vi "运维调试_总磷总氮.vi"() -> ()   [LabVIEW 2016, in "斯坦道仪器.lvlib"]
uses:
  <vilib>/Platform/TimedLoop/XDataNode/timing_clust.ctl
  <vilib>/Platform/TimedLoop/XDataNode/nitl_modes.ctl
  <vilib>/Platform/TimedLoop/XDataNode/wakeup.ctl
  <vilib>/Utility/miscctls.llb/LVPointTypeDef.ctl
  <vilib>/Utility/config.llb/Read Key (Double).vi
  <vilib>/Utility/config.llb/Write Key (Double).vi
  <vilib>/Platform/TimedLoop/XDataNode/XDataNode.xnode
  <vilib>/Platform/TimedLoop/XDataNode/XDNodeRunTimeDep.lvlib
  <vilib>/Utility/config.llb/NI_LVConfig.lvlib
panel:
  in  "返回 2":bool
  in  "设置 2":bool
  out "总氮稀释倍数":dbl
  out "固件版本号":string
  in  "数组":string[](array[string])
  in  "备用系数写入":bool
  in  "备用系数读取":bool
  in  "备用系数":T1
  in  "量程切换阈值写入":bool
  in  "量程切换阈值读取":bool
  in  "量程切换阈值":cluster{"阈值":dbl, "标液浓度":dbl}
  in  "参数下拉列表":enum16{"总磷", "总氮"}(ring)
  in  "量程下拉列表":enum16{"低量程", "高量程"}(ring)
  in  "测量模式下拉列表":enum16{"水样测量", "空白核查", "跨度核查", "标样核查", "加标回收"}(ring)
  in  "公式":cluster{"X^2":dbl, "X":dbl, "b":dbl}
  in  "写公式":bool
  in  "读公式":bool
  in  "精度":dbl=4.0
  in  "样品5 F0":dbl
  in  "样品5 F1":dbl
  in  "样品4 F1":dbl
  in  "样品4 F0":dbl
  in  "样品3 F0":dbl
  in  "样品3 F1":dbl
  in  "样品2 F0":dbl
  in  "样品2 F1":dbl
  in  "样品1 F1":dbl
  in  "样品1 F0":dbl
  in  "method":u16(ring) items=["最小二乘", "最小绝对残差", "Bisquare"]
  in  "模型":enum32{"线性", "多项式"}(ring)
  out "r^2":dbl format="%.7g"
  out "拟合公式":string
  in  "样品2启用":bool
  in  "样品5启用":bool
  in  "样品4启用":bool
  in  "样品3启用":bool
  in  "样品1启用":bool
  in  "标液浓度5":dbl
  in  "测量吸光度5":dbl
  in  "标液浓度4":dbl
  in  "测量吸光度4":dbl
  in  "标液浓度3":dbl
  in  "测量吸光度3":dbl
  in  "标液浓度2":dbl
  in  "测量吸光度2":dbl
  in  "测量吸光度1":dbl
  in  "标液浓度1":dbl
  out "XY图":cluster{"X Values":dbl[], "Y Values":dbl[]}[](graph)
  in  "返回":bool
  in  "调试":bool
  out "序列号":string="序列号"
  out "总氮测量数据":T2(xcontrol)
  out "总磷测量数据":T2(xcontrol)
  out "集成报警信息":string
  out "设置值":dbl
  out "定时启动":bool
  out "总磷总氮运行状态":T3(xcontrol)
  in  "停止":bool
  in  "手动启动":bool
  in  "单步测试":bool
  in  "总磷氨氮调试":u16[](xcontrol)
  out "F3":sgl format="%#.6f"
  out "F2":sgl format="%#.6f"
  out "F1":sgl format="%#.6f"
  out "F0":sgl format="%#.6f"
  out "多列列表框":i32(listbox)
  # "COM5"
  # "参数设置"
  # "标液浓度"
  # "F0"
  # "F1"
  # "吸光值显示"
  # "辅\n助\n计\n算\n区"
  # "样品一"
  # "样品二"
  # "样品三"
  # "样品四"
  # "样品五"
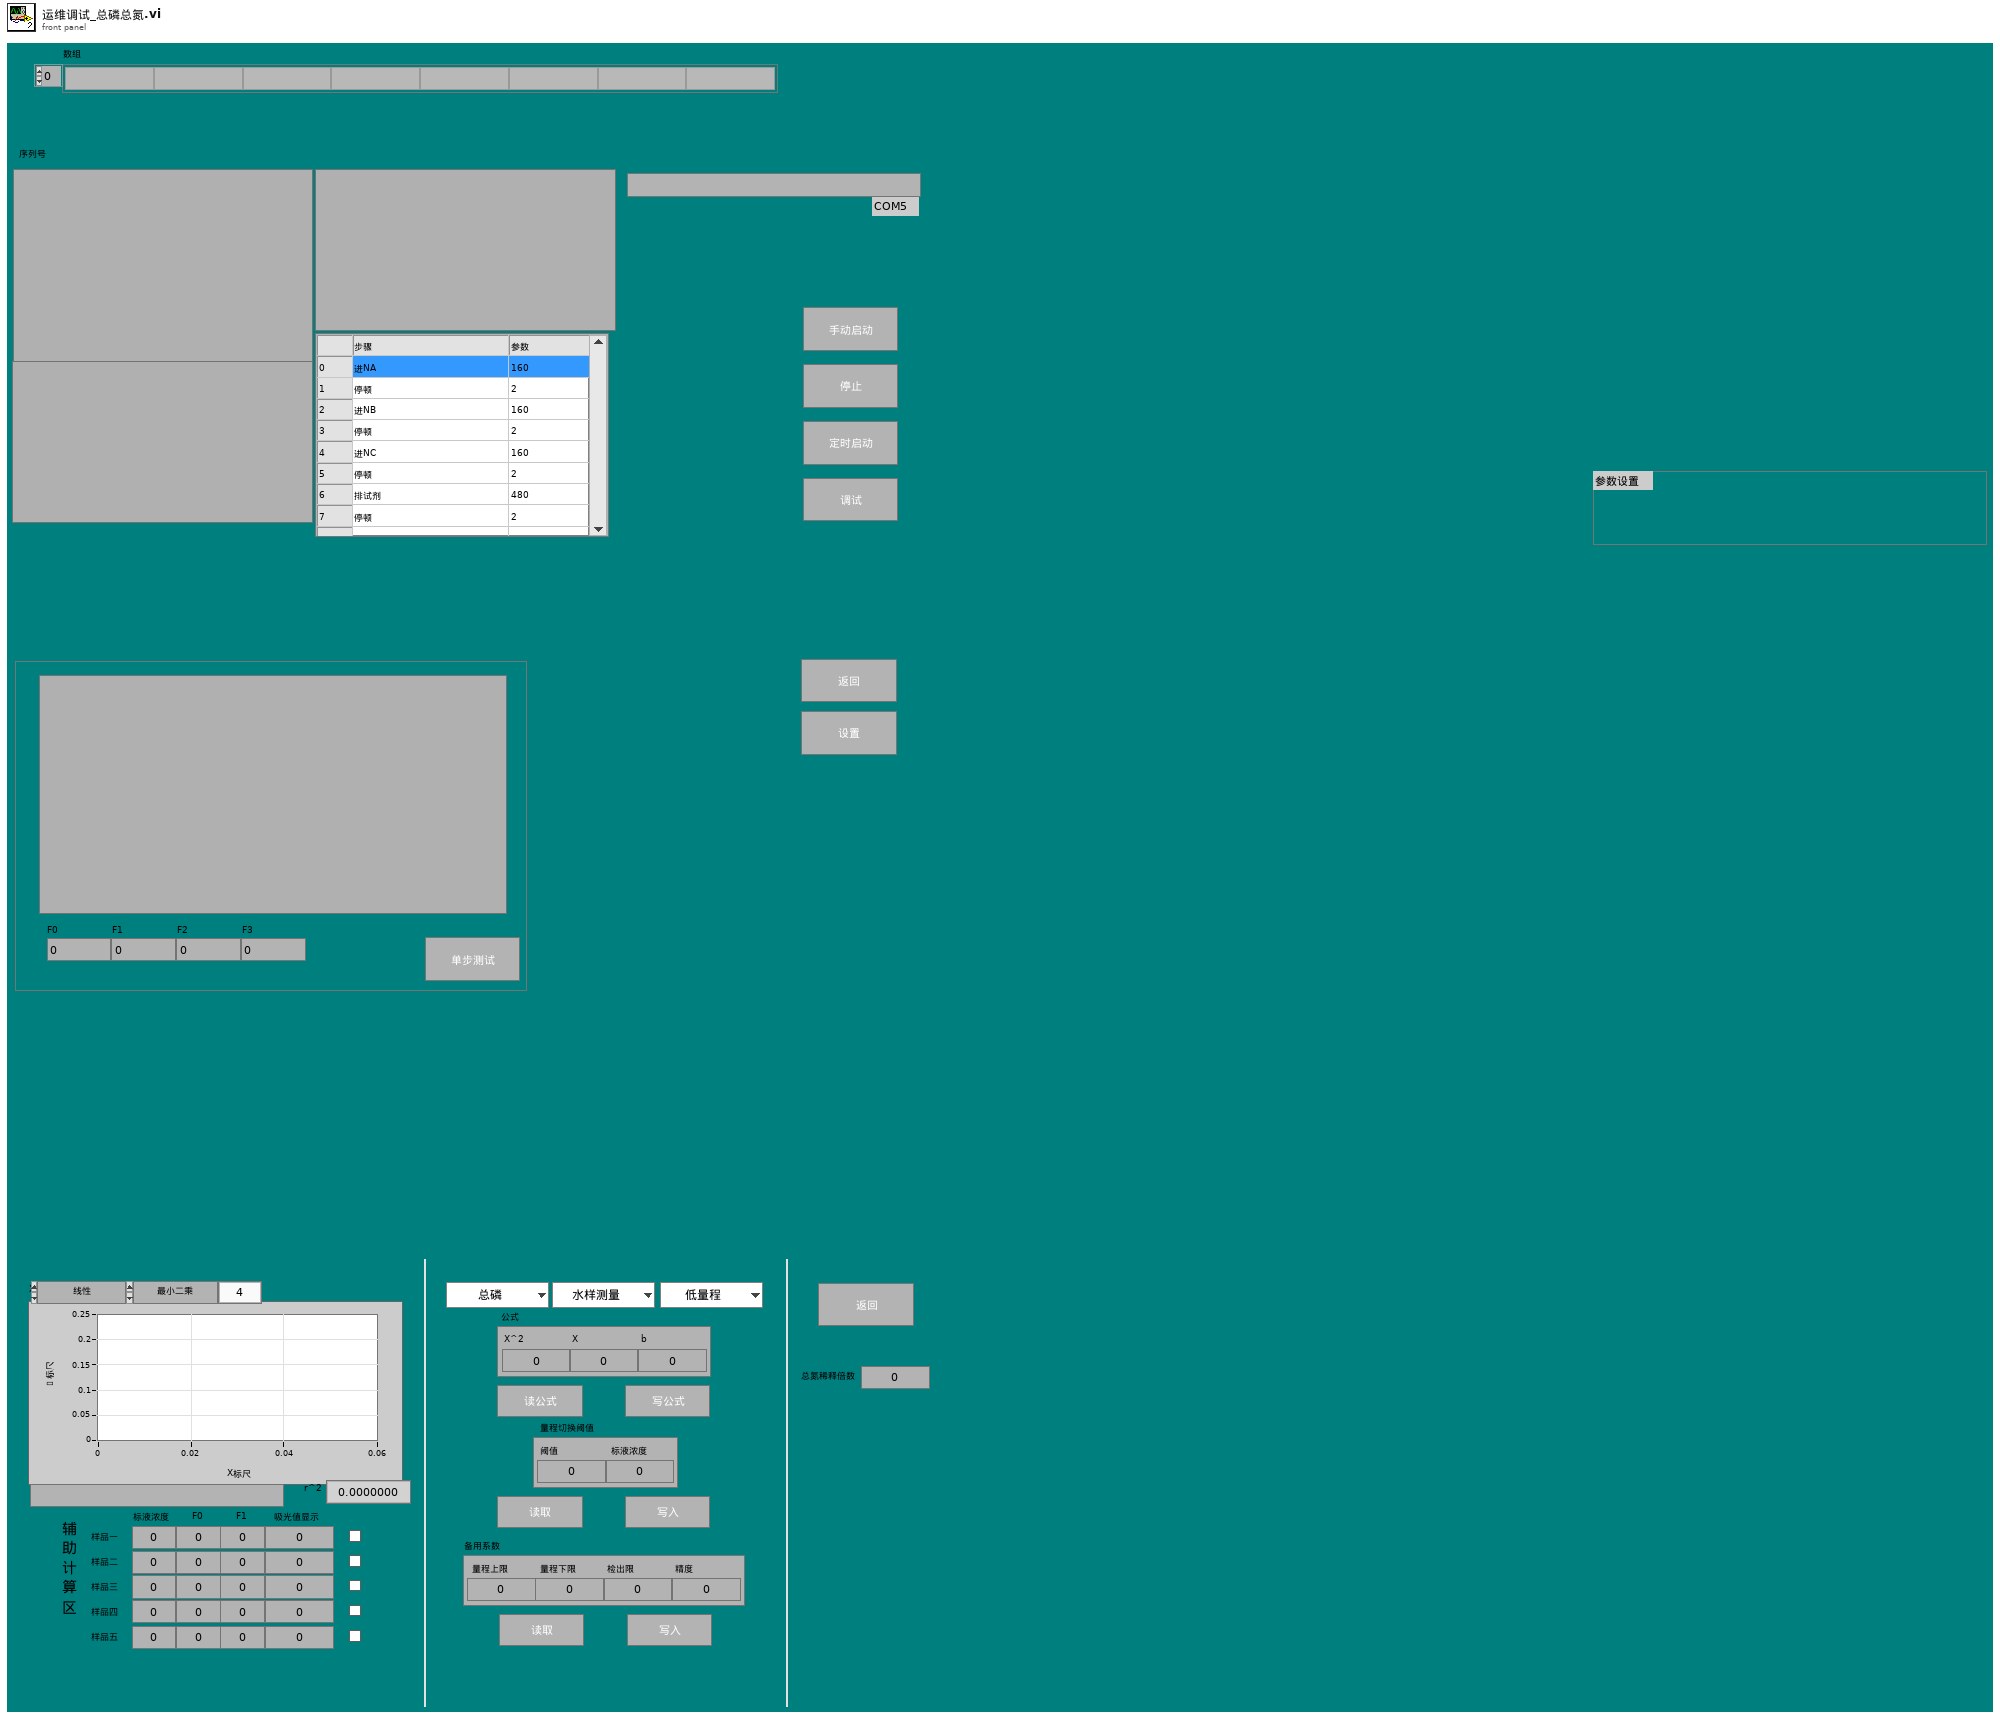
[diagram p1: front panel]
types:
  T1 = cluster{"量程上限":dbl, "量程下限":dbl, "检出限":dbl, "精度":dbl}
  T2 = cluster{"flowid":u16, "测量精度":u16, "测量数据区":cluster{"因子编码":u32, "单位":u16, "标样参考值":sgl, "水样数据时间":timestamp, "水样实测值":sgl, "水样数据标识":string, "标样数据时间":timestamp, "标样实测值":sgl, "标样数据标识":string, "空白数据时间":timestamp, "空白实测值":sgl, "空白数据标识":string, "零点核查数据时间":timestamp, "零点核查实测值":sgl, "零点核查数据标识":string, "跨度核查数据时间":timestamp, "跨度核查实测值":sgl, "跨度核查数据标识":string, "加标回收数据时间":timestamp, "加标回收实测值":sgl, "加标回收数据标识":string, "平行样数据时间":timestamp, "平行样实测值":sgl, "平行样数据标识":string, "F0":sgl, "F1":sgl, "F2":sgl, "F3":sgl, "F4":sgl, "F5":sgl, "F6":sgl, "F7":sgl, "温度":sgl, "湿度":sgl, "X值":sgl}}
  T3 = cluster{"系统时间":timestamp, "工作状态":enum16{"空闲", "水样测试", "标样核查", "零点核查", "跨度核查", "空白测试", "平行样测试", "加标回收", "空白校准", "标样校准", "初始化（清洗）"}, "测量模式":enum16{"待机", "连续模式", "周期模式", "定点模式", "受控模式", "手动模式"}, "告警代码":enum16{"无告警", "缺试剂告警", "缺水样告警", "缺蒸馏水告警", "缺标液告警", "仪表漏液告警", "标定异常告警", "超量程告警", "加热异常", "低试剂预警", "超上限告警", "超下限告警", "仪表内部其他异常", "滴定异常告警", "电极异常告警", "量程切换告警", "参数设置告警", "PH电极电位异常", "电导率电极异常", "浊度光度异常", "溶解氧电极异常", "溶解氧光强异常", "温度异常告警", "PH异常告警", "溶解氧异常告警", "电导率异常告警", "浊度异常告警", "叶绿素异常告警", "藻密度异常告警", "蓝绿藻异常告警", "ORP异常告警", "氨氮异常告警", "清洁刷异常告警", "SD卡异常告警", "蓝牙异常告警", "Wifi异常告警", "流程异常告警"}, "故障代码":enum16{"无故障", "电机故障", "温度故障", "通讯故障", "滴定故障"}, "日志代码":u16, "软件版本":u16, "F0":sgl, "F1":sgl, "F2":sgl, "F3":sgl, "T":sgl, "H":sgl, "id":u16, "flowid":u16, "量程":u16}
  T4 = enum16{"待机", "启动氨氮", "氨氮测量中", "启动总磷", "总磷测量中", "延时"}
  T5 = typedef "LVPointTypeDef.ctl" = cluster{"Horizontal":i16, "Vertical":i16}
  T6 = cluster{"因子编码":u32, "单位":u16, "标样参考值":sgl, "水样数据时间":timestamp, "水样实测值":sgl, "水样数据标识":string, "标样数据时间":timestamp, "标样实测值":sgl, "标样数据标识":string, "空白数据时间":timestamp, "空白实测值":sgl, "空白数据标识":string, "零点核查数据时间":timestamp, "零点核查实测值":sgl, "零点核查数据标识":string, "跨度核查数据时间":timestamp, "跨度核查实测值":sgl, "跨度核查数据标识":string, "加标回收数据时间":timestamp, "加标回收实测值":sgl, "加标回收数据标识":string, "平行样数据时间":timestamp, "平行样实测值":sgl, "平行样数据标识":string, "F0":sgl, "F1":sgl, "F2":sgl, "F3":sgl, "F4":sgl, "F5":sgl, "F6":sgl, "F7":sgl, "温度":sgl, "湿度":sgl, "X值":sgl}
  T7 = enum16{"空闲", "水样测试", "标样核查", "零点核查", "跨度核查", "空白测试", "平行样测试", "加标回收", "空白校准", "标样校准", "初始化（清洗）"}
  T8 = typedef "XDNodeRunTimeDep.lvlib/timing_clust.ctl" = cluster{"Expected End [f-1]":u64, "Actual End [f-1]":u64, "Finished Late? [f-1]":bool, "Expected End [i-1]":u64, "Actual End [i-1]":u64, "Finished Late? [i-1]":bool, "Expected Start [i]":u64, "Actual Start [i]":u64, "Expected Start [f]":u64, "Actual Start [f]":u64, "Source Name":string, "Structure Name":string, "Period":i64, "Deadline":i64, "Offset":i64, "Start":i64, "Priority":i32, "Timeout":i32, "Mode":T9, "Wakeup Reason":T10, "Error":errorcluster, "Source Type":string, "Secondary Source Type":string, "Global End Time":u64, "Global Start Time":u64, "Frame Duration":u64, "Iteration Duration":u64, "Assigned CPU":i32, "I/O Scan Engine Mode":u32}
  T9 = typedef "XDNodeRunTimeDep.lvlib/nitl_modes.ctl" = enum32{"No Change", "Process missed periods, maintain original phase", "Discard missed periods, maintain original phase", "Process missed periods, ignore original phase", "Discard missed periods, ignore original phase"}
  T10 = typedef "XDNodeRunTimeDep.lvlib/wakeup.ctl" = enum32{"Normal", "Aborted", "Asynchronous wakeup", "Timing source error", "Timed loop error", "Timeout"}
  T11 = cluster{"启动模式":enum16{"标液测量", "水样测量", "零液测量", "盲样测量", "加标回收"}, "启动参数":u16, "量程":enum16{"低量程", "高量程"}}
  T12 = cluster{"时间标识":timestamp, "设备":string, "日志信息":string, "流程参数":string}
  T13 = cluster{"时间标识":timestamp, "设备":string, "日志信息":string}
  T14 = enum16{"无告警", "缺试剂告警", "缺水样告警", "缺蒸馏水告警", "缺标液告警", "仪表漏液告警", "标定异常告警", "超量程告警", "加热异常", "低试剂预警", "超上限告警", "超下限告警", "仪表内部其他异常", "滴定异常告警", "电极异常告警", "量程切换告警", "参数设置告警", "PH电极电位异常", "电导率电极异常", "浊度光度异常", "溶解氧电极异常", "溶解氧光强异常", "温度异常告警", "PH异常告警", "溶解氧异常告警", "电导率异常告警", "浊度异常告警", "叶绿素异常告警", "藻密度异常告警", "蓝绿藻异常告警", "ORP异常告警", "氨氮异常告警", "清洁刷异常告警", "SD卡异常告警", "蓝牙异常告警", "Wifi异常告警", "流程异常告警"}
  T15 = typedef "LVRowAndColumnUnsignedTypeDef.ctl" = cluster{"Row":u32, "Column":u32}
  T16 = typedef "NI_LVConfig.lvlib/Config Data RefNum.ctl" = refnum<k1>
  T17 = cluster{"站号":u16, "量程切换":enum32{"H", "L", "AUTO"}, "控制命令":enum16{"启动测量", "标样核查", "零点核查", "跨度核查", "空白测试", "平行样测试", "加标回收", "空白校准", "标样校准", "初始化（清洗）", "停止测试", "仪器重启", "校时", "模式设置", "测量间隔设置", "盲样测试"}, "模式设置":enum16{"待机", "连续模式", "周期模式", "定点模式", "受控模式", "手动模式"}, "测量间隔":u16}
  T18 = cluster{"站号":u16, "量程切换":enum32{"H", "L", "AUTO"}, "控制命令":enum16{"启动测量", "标样核查", "零点核查", "跨度核查", "空白测试", "平行样测试", "加标回收", "空白校准", "标样校准", "初始化（清洗）", "停止测试", "仪器重启", "校时", "模式设置", "测量间隔设置"}, "模式设置":enum16{"待机", "连续模式", "周期模式", "定点模式", "受控模式", "手动模式"}, "测量间隔":u16}
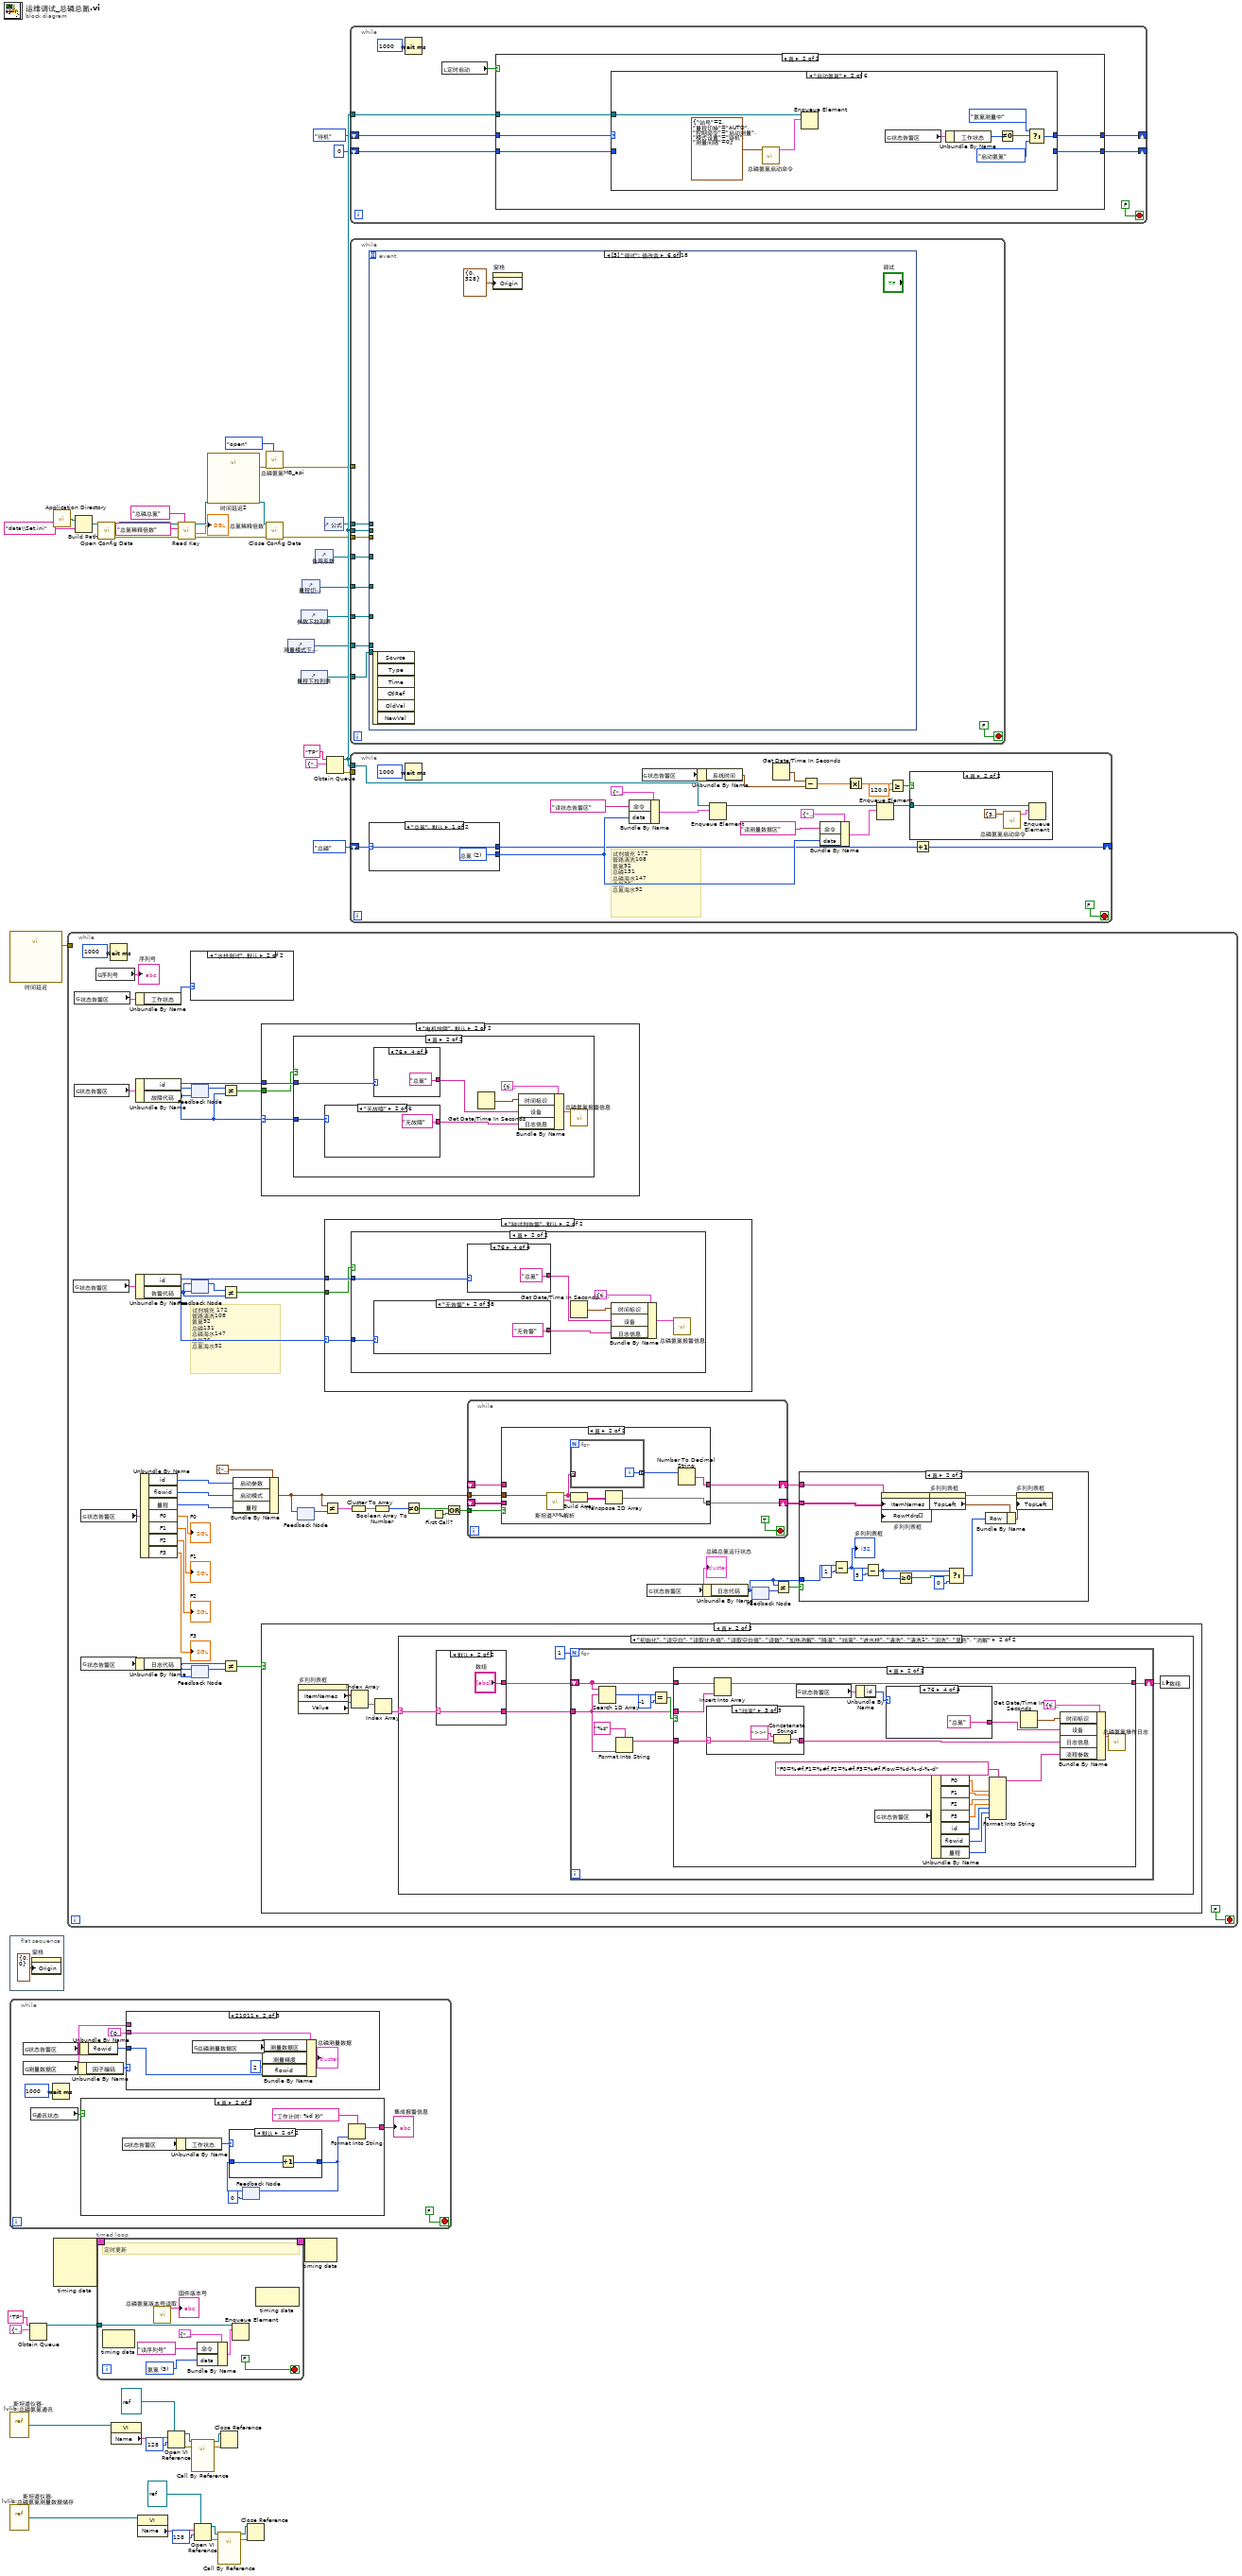
[diagram p0: block diagram]
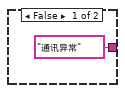
[diagram p2: hidden frame]
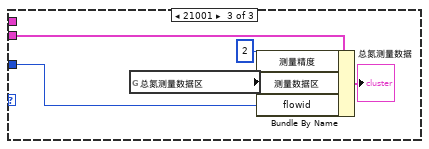
[diagram p5: hidden frame]
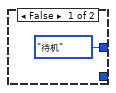
[diagram p6: hidden frame]
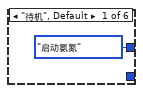
[diagram p7: hidden frame]
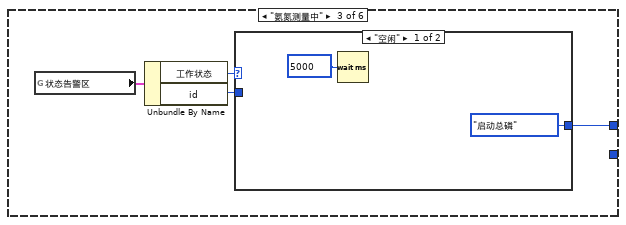
[diagram p8: hidden frame]
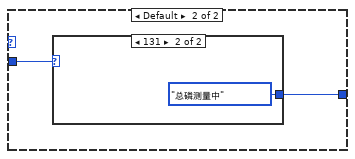
[diagram p9: hidden frame]
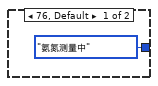
[diagram p10: hidden frame]
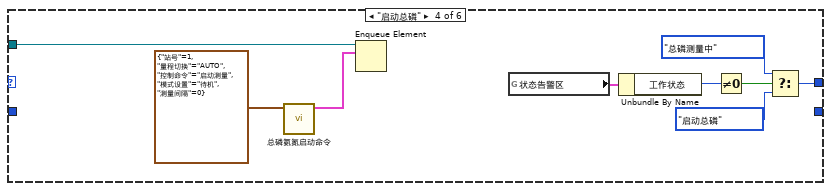
[diagram p11: hidden frame]
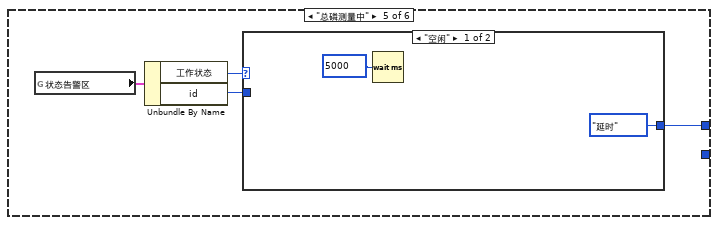
[diagram p12: hidden frame]
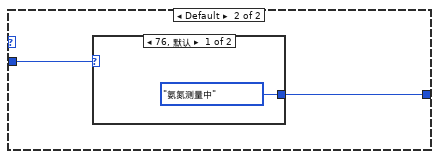
[diagram p13: hidden frame]
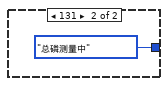
[diagram p14: hidden frame]
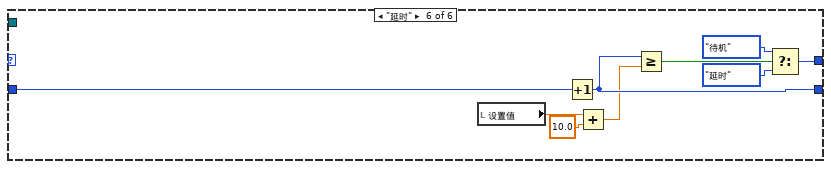
[diagram p15: hidden frame]
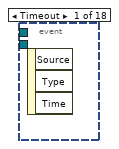
[diagram p16: hidden frame]
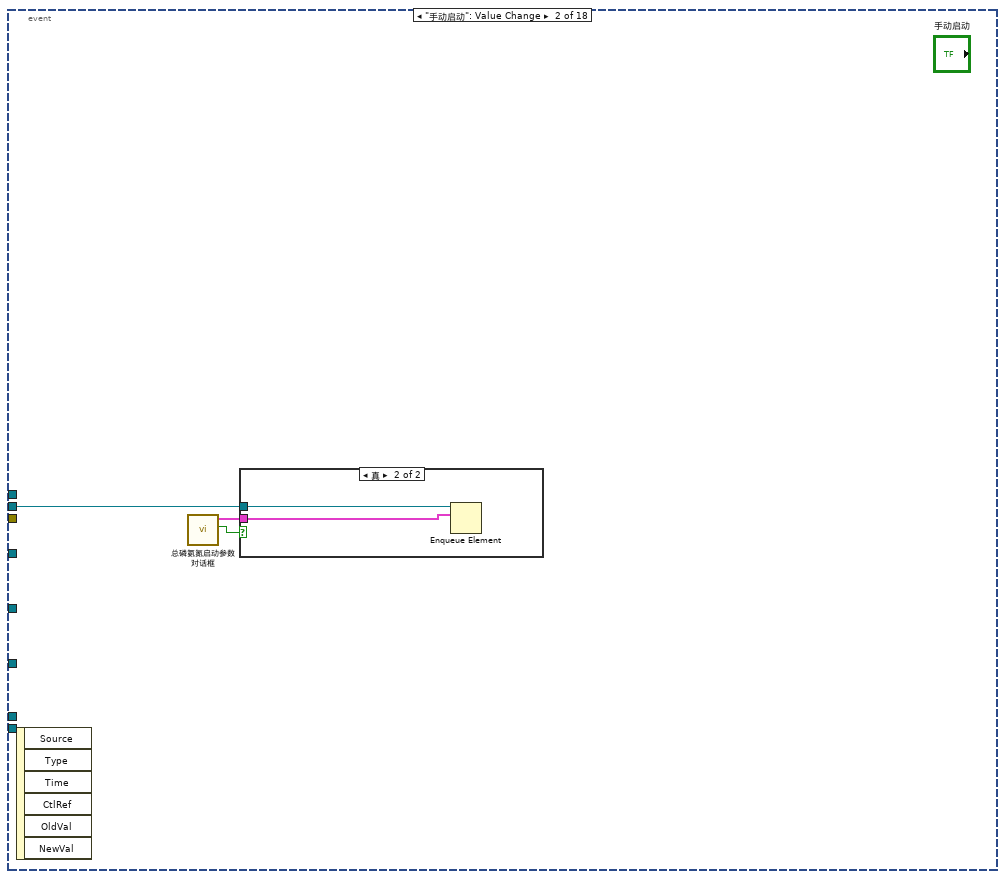
[diagram p17: hidden frame]
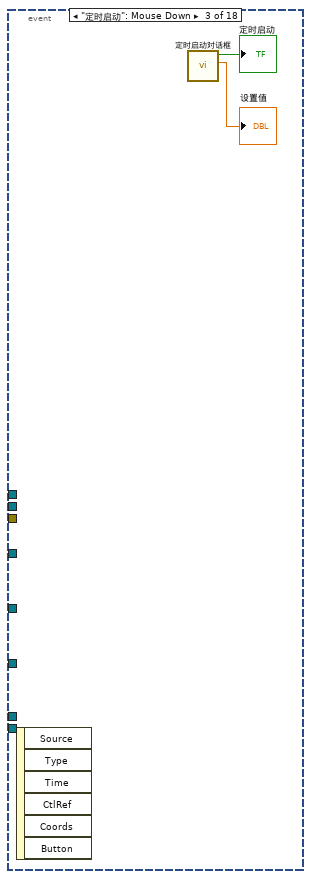
[diagram p19: hidden frame]
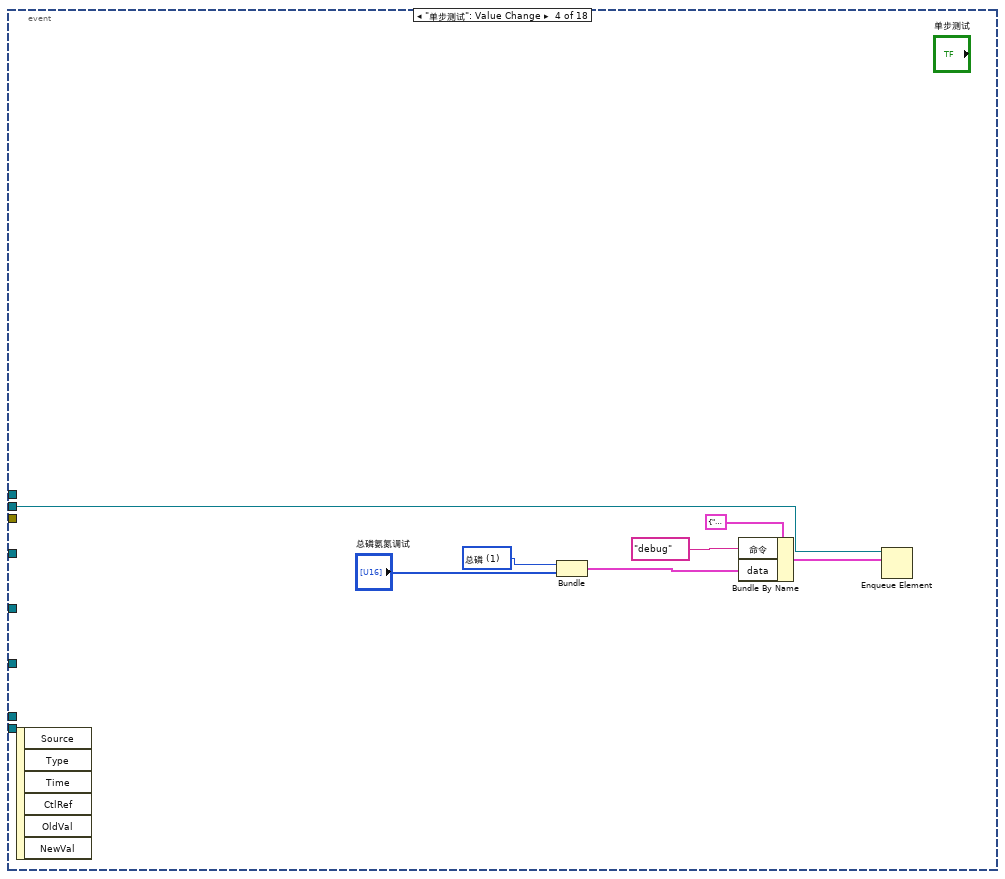
[diagram p20: hidden frame]
diagram:
  n1 = call "时间延迟"() -> ("error out"=w20:errorcluster)  [unwired: 11 in]
  n2 = flat-sequence {
    frame #0 {
      n3 = property on="窗格" class="Pane"("Origin"=T5 {"Horizontal"=0, "Vertical"=0} ("原点")) -> ()  [unwired: 2 in, 2 out]
    }
  }
  n4 = while {
    stop <- FALSE stop-if-true
    n5 = global read "VAR总磷氨氮全局变量.vi" "状态告警区"() -> (w53:T3)
    n6 = global read "VAR总磷氨氮全局变量.vi" "测量数据区"() -> (w57:T6)
    n7 = global read "VAR总磷氨氮全局变量.vi" "通讯状态"() -> (w55:bool)
    n8 = Wait (ms)(milliseconds to wait=u32 1000 ("等待时间（毫秒）")) -> ()  [unwired: 1 out]
    n9 = Unbundle By Name(w57) -> ("因子编码"=w56:u32)
    n10 = Unbundle By Name(w53) -> ("flowid"=w52:u16)
    n11 = case shown="真" w55 {
      tunnel: ["通讯异常" ("集成报警信息") w61] -> w54
      frame False {
      }
      frame True {
        n12 = global read "VAR总磷氨氮全局变量.vi" "状态告警区"() -> (w67:T3)
        n13 = Unbundle By Name(w67) -> ("工作状态"=w66:T7)
        n14 = feedback #1(0) -> (w64:i32)
        n15 = case shown="默认" w66 {
          tunnel: w64 -> [_ w69]
          tunnel: [_ w68] -> w62
          frame "空闲" {
          }
          frame Default {
            n16 = Increment(x=w69) -> (x+1=w68:i32)
          }
        }
        n17 = feedback-in #1(w62) -> ()
        n18 = Format Into String(format string="工作计时: %d 秒" ("格式字符串"), w62) -> (resulting string=w61:string)  [unwired: 2 in, 1 out]
      }
    }
    "集成报警信息" <- w54
    n19 = case shown="21011" w56 {
      tunnel: w57 -> [_ _ _]
      tunnel: w52 -> [_ w72 w78]
      tunnel: T2 {"flowid"=0, "测量精度"=0, "测量数据区"={"因子编码"=0, "单位"=0, "标样参考值"=0.0, "水样数据时间"=timestamp(0 s since 1904-01-01), "水样实测值"=0.0, "水样数据标识"="", "标样数据时间"=timestamp(0 s since 1904-01-01), "标样实测值"=0.0, "标样数据标识"="", "空白数据时间"=timestamp(0 s since 1904-01-01), "空白实测值"=0.0, "空白数据标识"="", "零点核查数据时间"=timestamp(0 s since 1904-01-01), "零点核查实测值"=0.0, "零点核查数据标识"="", "跨度核查数据时间"=timestamp(0 s since 1904-01-01), "跨度核查实测值"=0.0, "跨度核查数据标识"="", "加标回收数据时间"=timestamp(0 s since 1904-01-01), "加标回收实测值"=0.0, "加标回收数据标识"="", "平行样数据时间"=timestamp(0 s since 1904-01-01), "平行样实测值"=0.0, "平行样数据标识"="", "F0"=0.0, "F1"=0.0, "F2"=0.0, "F3"=0.0, "F4"=0.0, "F5"=0.0, "F6"=0.0, "F7"=0.0, "温度"=0.0, "湿度"=0.0, "X值"=0.0}} ("总氮测量数据") -> [_ w71 w77]
      frame Default {
      }
      frame 21011 {
        n20 = global read "VAR总磷氨氮全局变量.vi" "总磷测量数据区"() -> (w70:T6)
        n21 = Bundle By Name(cluster=w71, "测量数据区"=w70, "测量精度"=u16 2, "flowid"=w72) -> (→"总磷测量数据":T2)
      }
      frame 21001 {
        n22 = global read "VAR总磷氨氮全局变量.vi" "总氮测量数据区"() -> (w75:T6)
        n23 = Bundle By Name(cluster=w77, "测量精度"=u16 2, "测量数据区"=w75, "flowid"=w78) -> (→"总氮测量数据":T2)
      }
    }
  }
  n24 = vi-ref "斯坦道仪器.lvlib:总磷氨氮通讯.vi"() -> (w43:refnum<vi>)
  n25 = vi-ref "斯坦道仪器.lvlib:总磷氨氮测量数据储存.vi"() -> (w35:refnum<vi>)
  n26 = Obtain Queue(name (unnamed)="TP" ("名称（未命名）"), element data type=cluster{"命令":string, "data":variant} {"命令"="", "data"=variant}) -> (queue out=w13:refnum<queue>)  [unwired: 3 in, 2 out]
  n27 = node-c288() -> (w17:T8)  [unwired: 4 in]
  n28 = call <vilib>:"Application Directory.vi"() -> ("Application Directory"=w7:path)
  n29 = while {
    tunnel: w20 -> [_]
    stop <- FALSE stop-if-true
    # "试剂填充 172 \n管路清洗108\n氨氮92\n总磷131\n总磷海水147\n总氮76\n总氮海水92"
    n30 = global read "VAR总磷氨氮全局变量.vi" "状态告警区"() -> (w96:T3)
    n31 = global read "VAR总磷氨氮全局变量.vi" "状态告警区"() -> (w91:T3)
    n32 = global read "VAR总磷氨氮全局变量.vi" "状态告警区"() -> (w85:T3)
    n33 = global read "VAR总磷氨氮全局变量.vi" "状态告警区"() -> (w108:T3)
    n34 = global read "VAR总磷氨氮全局变量.vi" "状态告警区"() -> (w82:T3)
    n35 = global read "VAR总磷氨氮全局变量.vi" "序列号"() -> (→"序列号":string)
    n36 = Wait (ms)(milliseconds to wait=u32 1000 ("等待时间（毫秒）")) -> ()  [unwired: 1 out]
    n37 = Unbundle By Name(w85) -> ("工作状态"=w84:T7)
    n38 = Unbundle By Name(w91) -> ("id"=w90:u16, "故障代码"=w87:enum16{"无故障", "电机故障", "温度故障", "通讯故障", "滴定故障"})
    n39 = Unbundle By Name(w96) -> ("id"=w95:u16, "告警代码"=w92:T14)
    n40 = Unbundle By Name(w82) -> ("日志代码"=w81:u16)
    n41 = Unbundle By Name(w108) -> ("id"=w105:u16, "flowid"=w107:u16, "量程"=w106:u16, "F0"=→"F0":sgl, "F1"=→"F1":sgl, "F2"=→"F2":sgl, "F3"=→"F3":sgl)
    n42 = case shown="\"水样测试\", 默认" w84 {
      frame "空闲" {
        n43 = local write "数组"(string[] [] ("数组")) -> ()
      }
      frame "水样测试", Default {
      }
    }
    n44 = feedback #2(w87) -> (w88:enum16{"无故障", "电机故障", "温度故障", "通讯故障", "滴定故障"})
    n45 = feedback-in #2(w87) -> ()
    n46 = feedback #3(w92) -> (w93:T14)
    n47 = feedback-in #3(w92) -> ()
    n48 = feedback #4(w81) -> (w83:u16)
    n49 = feedback-in #4(w81) -> ()
    n50 = Not Equal?(x=w88, y=w87) -> (x != y?=w89:bool)
    n51 = Not Equal?(x=w93, y=w92) -> (x != y?=w94:bool)
    n52 = Not Equal?(x=w81, y=w83) -> (x != y?=w80:bool)
    n53 = Bundle By Name(cluster=T11 {"启动模式"=enum."加标回收", "启动参数"=1, "量程"=enum."低量程"} ("参数簇"), "启动参数"=w105, "启动模式"=w107, "量程"=w106) -> (w98:T11)
    n54 = case shown="\"电机故障\", 默认" w87 {
      selector: w87 -> [_ w177]
      tunnel: w90 -> [_ w178]
      tunnel: w89 -> [_ w176]
      frame "无故障" {
      }
      frame "电机故障", Default {
        n55 = case shown="真" w176 {
          tunnel: w178 -> [_ w185]
          tunnel: w177 -> [_ w180]
          frame False {
          }
          frame True {
            n56 = case shown="\"无故障\"" w180 {
              selector: w180 -> [w187 _ _ _ _ _]
              tunnel: [w186 "无故障" "电机故障" "温度故障" "通讯故障" "滴定故障"] -> w179
              frame Default {
                n57 = Format Into String(format string="%d" ("格式字符串"), initial string="未知" ("工作状态"), w187) -> (resulting string=w186:string)  [unwired: 1 in, 1 out]
              }
              frame "无故障" {
              }
              frame "电机故障" {
              }
              frame "温度故障" {
              }
              frame "通讯故障" {
              }
              frame "滴定故障" {
              }
            }
            n58 = case shown="76" w185 {
              tunnel: [_ "总磷" ("table输入") "氨氮" ("table输入") "总氮" ("table输入")] -> w181
              frame Default {
              }
              frame 131 {
              }
              frame 92 {
              }
              frame 76 {
              }
            }
            n59 = Get Date/Time In Seconds() -> (seconds since 1Jan1904=w182:timestamp)
            n60 = Bundle By Name(cluster=T13 {"时间标识"=timestamp(0 s since 1904-01-01), "设备"="", "日志信息"=""} ("data in"), "时间标识"=w182, "设备"=w181, "日志信息"=w179) -> (w183:T13)
            n61 = call "总磷氨氮报警信息.vi"("data in"=w183) -> ()  [unwired: 11 in]
          }
        }
      }
    }
    n62 = case shown="真" w80 {
      frame False {
      }
      frame True {
        n63 = property on="多列列表框" class="MCListbox (严格)"() -> ("ItemNames"=w125:string[][], "Value"=w126:i32)  [unwired: 2 in, 2 out]
        n64 = Index Array(array=w125, index (row)=w126) -> (element=w124:string[])  [unwired: 1 in]
        n65 = Index Array(array=w124) -> (element=w123:string)  [unwired: 1 in]
        n66 = case shown="\"初始化\", \"读空白\", \"读取比色值\", \"读取空白值\", \"读数\", \"加热消解\", \"降温\", \"结束\", \"进水样\", \"清洗\", \"清洗1\", \"润洗\", \"显色\", \"消解\"" w123 {
          selector: w123 -> [_ w129]
          frame Default {
          }
          frame "初始化", "读空白", "读取比色值", "读取空白值", "读数", "加热消解", "降温", "结束", "进水样", "清洗", "清洗1", "润洗", "显色", "消解" {
            n67 = case shown="默认" w129 {
              selector: w129 -> [w133 w135]
              tunnel: [w133 w135] -> w128
              tunnel: [string[] [] ("数组") "数组"] -> w127
              frame "读数" {
              }
              frame Default {
              }
            }
            n68 = for {
              N: 1 -> [_]
              tunnel: w128 -> [w137]
              shift-right: [w136] -> w130
              shift-left: w127 -> [w138]
              n69 = Search 1D Array(1D array=w138, element=w137) -> (index of element=w141:i32)  [unwired: 1 in]
              n70 = Format Into String(format string="%s" ("格式字符串"), w137) -> (resulting string=w142:string)  [unwired: 2 in, 1 out]
              n71 = Equal?(x=w141, y=-1) -> (x = y?=w139:bool)
              n72 = case shown="真" w139 {
                tunnel: w142 -> [_ w146]
                tunnel: w138 -> [w144 w150]
                tunnel: w137 -> [_ w149]
                tunnel: [w144 w148] -> w136
                frame False {
                }
                frame True {
                  n73 = case shown="\"结束\"" w146 {
                    selector: w146 -> [w166 w169 w172]
                    tunnel: [w166 w168 w171] -> w145
                    frame Default {
                    }
                    frame "初始化" {
                      n74 = Concatenate Strings("<<" ("字符串"), w169) -> (w168:string)
                    }
                    frame "结束" {
                      n75 = Concatenate Strings(">>" ("字符串"), w172) -> (w171:string)
                    }
                  }
                  n76 = Insert Into Array(array=w150, new element=w149) -> (w148:string[])  [unwired: 1 in]
                  n77 = global read "VAR总磷氨氮全局变量.vi" "状态告警区"() -> (w165:T3)
                  n78 = Unbundle By Name(w165) -> ("id"=w164:u16)
                  n79 = global read "VAR总磷氨氮全局变量.vi" "状态告警区"() -> (w160:T3)
                  n80 = case shown="76" w164 {
                    tunnel: [_ "总磷" ("table输入") "氨氮" ("table输入") "总氮" ("table输入")] -> w162
                    frame Default {
                    }
                    frame 131 {
                    }
                    frame 92 {
                    }
                    frame 76 {
                    }
                  }
                  n81 = Unbundle By Name(w160) -> ("F0"=w157:sgl, "F1"=w156:sgl, "F2"=w155:sgl, "F3"=w154:sgl, "id"=w153:u16, "flowid"=w152:u16, "量程"=w151:u16)
                  n82 = Format Into String(format string="F0=%#f,F1=%#f,F2=%#f,F3=%#f,Flow=%d-%-d-%-d" ("格式字符串"), w157, w156, w155, w154, w153, w152, w151) -> (resulting string=w158:string)  [unwired: 2 in, 1 out]
                  n83 = Get Date/Time In Seconds() -> (seconds since 1Jan1904=w161:timestamp)
                  n84 = Bundle By Name(cluster=T12 {"时间标识"=timestamp(0 s since 1904-01-01), "设备"="", "日志信息"="", "流程参数"=""} ("data in"), "时间标识"=w161, "设备"=w162, "日志信息"=w145, "流程参数"=w158) -> (w163:T12)
                  n85 = call "总磷氨氮操作日志.vi"("data in"=w163) -> ()  [unwired: 11 in]
                }
              }
            }
            n86 = local write "数组"(w130) -> ()
          }
        }
      }
    }
    n87 = feedback #5() -> (w114:T11)  [unwired: 1 in]
    n88 = feedback-in #5(w98) -> ()
    n89 = Not Equal?(x=w98, y=w114) -> (x != y?=w115:cluster{"启动模式":bool, "启动参数":bool, "量程":bool})
    n90 = case shown="\"缺试剂告警\", 默认" w92 {
      selector: w92 -> [_ w199]
      tunnel: w95 -> [_ w200]
      tunnel: w94 -> [_ w198]
      frame "无告警" {
      }
      frame "缺试剂告警", Default {
        n91 = case shown="真" w198 {
          tunnel: w200 -> [_ w207]
          tunnel: w199 -> [_ w201]
          frame False {
          }
          frame True {
            n92 = case shown="\"无告警\"" w201 {
              selector: w201 -> [w209 _ _ _ _ _ _ _ _ _ _ _ _ _ _ _ _ _ _ _ _ _ _ _ _ _ _ _ _ _ _ _ _ _ _ _ _ _]
              tunnel: [w208 "无告警" "缺试剂告警" "缺水样告警" "缺蒸馏水告警" "缺标液告警" "仪表漏液告警" "标定异常告警" "超量程告警" "加热异常" "低试剂预警" "超上限告警" "超下限告警" "仪表内部其他异常" "滴定异常告警" "电极异常告警" "量程切换告警" "参数设置告警" "PH电极电位异常" "电导率电极异常" "浊度光度异常" "溶解氧电极异常" "溶解氧光强异常" "温度异常告警" "PH异常告警" "溶解氧异常告警" "电导率异常告警" "浊度异常告警" "叶绿素异常告警" "藻密度异常告警" "蓝绿藻异常告警" "ORP异常告警" "氨氮异常告警" "清洁刷异常告警" "SD卡异常告警" "蓝牙异常告警" "WiFi异常告警" "流程异常告警"] -> w202
              frame Default {
                n93 = Format Into String(format string="%d" ("格式字符串"), initial string="未知" ("工作状态"), w209) -> (resulting string=w208:string)  [unwired: 1 in, 1 out]
              }
              frame "无告警" {
              }
              frame "缺试剂告警" {
              }
              frame "缺水样告警" {
              }
              frame "缺蒸馏水告警" {
              }
              frame "缺标液告警" {
              }
              frame "仪表漏液告警" {
              }
              frame "标定异常告警" {
              }
              frame "超量程告警" {
              }
              frame "加热异常" {
              }
              frame "低试剂预警" {
              }
              frame "超上限告警" {
              }
              frame "超下限告警" {
              }
              frame "仪表内部其他异常" {
              }
              frame "滴定异常告警" {
              }
              frame "电极异常告警" {
              }
              frame "量程切换告警" {
              }
              frame "参数设置告警" {
              }
              frame "PH电极电位异常" {
              }
              frame "电导率电极异常" {
              }
              frame "浊度光度异常" {
              }
              frame "溶解氧电极异常" {
              }
              frame "溶解氧光强异常" {
              }
              frame "温度异常告警" {
              }
              frame "PH异常告警" {
              }
              frame "溶解氧异常告警" {
              }
              frame "电导率异常告警" {
              }
              frame "浊度异常告警" {
              }
              frame "叶绿素异常告警" {
              }
              frame "藻密度异常告警" {
              }
              frame "蓝绿藻异常告警" {
              }
              frame "ORP异常告警" {
              }
              frame "氨氮异常告警" {
              }
              frame "清洁刷异常告警" {
              }
              frame "SD卡异常告警" {
              }
              frame "蓝牙异常告警" {
              }
              frame "Wifi异常告警" {
              }
              frame "流程异常告警" {
              }
            }
            n94 = case shown="76" w207 {
              tunnel: [_ "总磷" ("table输入") "氨氮" ("table输入") "总氮" ("table输入")] -> w203
              frame Default {
              }
              frame 131 {
              }
              frame 92 {
              }
              frame 76 {
              }
            }
            n95 = Get Date/Time In Seconds() -> (seconds since 1Jan1904=w204:timestamp)
            n96 = Bundle By Name(cluster=T13 {"时间标识"=timestamp(0 s since 1904-01-01), "设备"="", "日志信息"=""} ("data in"), "时间标识"=w204, "设备"=w203, "日志信息"=w202) -> (w205:T13)
            n97 = call "总磷氨氮报警信息.vi"("data in"=w205) -> ()  [unwired: 11 in]
          }
        }
      }
    }
    n98 = Cluster To Array(cluster=w115) -> (array=w116:bool[])
    n99 = Boolean Array To Number(Boolean array=w116) -> (number=w117:u32)
    n100 = Not Equal To 0?(x=w117) -> (x != 0?=w110:bool)
    n101 = First Call?() -> (First Call?: T/F=w111:bool)
    n102 = Or(x=w110, y=w111) -> (x .or. y?=w109:bool)
    n103 = while {
      tunnel: w109 -> [w258]
      tunnel: w98 -> [w257]
      shift-right: [w256] -> w113
      shift-left: _ -> [w252]
      shift-right: [w255] -> w112
      shift-left: _ -> [w253]
      stop <- TRUE stop-if-true
      n104 = case shown="真" w258 {
        tunnel: [w260 w267] -> w255
        tunnel: [w259 w266] -> w256
        tunnel: w257 -> [_ w261]
        tunnel: w253 -> [w260 _]
        tunnel: w252 -> [w259 _]
        frame False {
        }
        frame True {
          n105 = call "斯坦道XML解析.vi"("参数簇"=w261) -> ("步骤时间"=w262:string[], "步骤名"=w264:string[])  [unwired: 9 in]
          n106 = for {
            tunnel: w264 -> [_] mode=indexing
            tunnel: [w268] -> w265 mode=indexing
            i -> [w268]
          }
          n107 = Build Array(w264, w262) -> (w263:string[][])
          n108 = Transpose 2D Array(2D array=w263) -> (transposed array=w266:string[][])
          n109 = Number To Decimal String(number=w265) -> (decimal integer string=w267:string[])  [unwired: 1 in]
        }
      }
    }
    n110 = global read "VAR总磷氨氮全局变量.vi" "状态告警区"() -> (w99:T3)
    "总磷总氮运行状态" <- w99
    n111 = Unbundle By Name(w99) -> ("日志代码"=w86:u16)
    n112 = feedback-in #6(w86) -> ()
    n113 = feedback #6() -> (w119:u16)  [unwired: 1 in]
    n114 = Not Equal?(x=w86, y=w119) -> (x != y?=w118:bool)
    n115 = case shown="真" w118 {
      tunnel: w86 -> [_ w271]
      tunnel: w113 -> [_ w278]
      tunnel: w112 -> [_ w277]
      frame False {
      }
      frame True {
        n116 = Subtract(x=w271, y=1) -> (x-y=w269:i32)
        "多列列表框" <- w269
        n117 = Subtract(x=w269, y=5) -> (x-y=w273:i32)
        n118 = property on="多列列表框" class="MCListbox (严格)"("ItemNames"=w278, "RowHdrs[]"=w277) -> (error out=w279:errorcluster)  [unwired: 2 in, 1 out]
        n119 = Greater Or Equal To 0?(x=w273) -> (x >= 0?=w272:bool)
        n120 = property on="多列列表框" class="MCListbox (严格)"(error in=w279) -> (error out=w280:errorcluster, "TopLeft"=w281:T15)  [unwired: 1 in, 1 out]
        n121 = Select(t=w273, s=w272, f=0) -> (s? t:f=w274:i32)
        n122 = Bundle By Name(cluster=w281, "Row"=w274) -> (w282:T15)
        n123 = property on="多列列表框" class="MCListbox (严格)"(error in=w280, "TopLeft"=w282) -> ()  [unwired: 1 in, 2 out]
      }
    }
  }
  n124 = Build Path(base path=w7, name or relative path="data\\Set.ini" ("名称或相对路径")) -> (appended path=w5:path)
  n125 = timed-loop {
    timing: w17 -> [_]
    timing-out: [_] -> w16
    tunnel: w13 -> [w285]
    stop <- FALSE stop-if-true
    w286 = u16 3 items=["总磷"=1, "氨氮"=3] ("站号")
    # "定时更新"
    n126 = node-c288() -> ()  [unwired: 1 in, 1 out]
    n127 = call "总磷氨氮版本号读取.vi"() -> ("固件版本号"=→"固件版本号":string)  [unwired: 11 in]
    n128 = Bundle By Name(cluster=cluster{"命令":string, "data":variant} {"命令"="", "data"=variant} ("元素"), "命令"="读序列号", "data"=w286) -> (w284:cluster{"命令":string, "data":variant})
    n129 = Enqueue Element(queue=w285, element=w284) -> ()  [unwired: 2 in, 3 out]
    n130 = node-c288() -> ()  [unwired: 1 in, 1 out]
  }
  n131 = call <vilib>:"Open Config Data.vi"("configuration file path"=w5) -> ("error out"=w9:errorcluster, "refnum"=w11:T16)  [unwired: 8 in, 1 out]
  n132 = property class="VI"(reference=w43) -> ("Name"=w42:string)  [unwired: 1 in, 2 out]
  n133 = property class="VI"(reference=w35) -> ("Name"=w28:string)  [unwired: 1 in, 2 out]
  n134 = Open VI Reference(type specifier VI Refnum (for type only)=refnum<vi> refnum, vi path=w42, options=128 ("选项")) -> (vi reference=w40:refnum<vi>, error out=w38:errorcluster)  [unwired: 3 in]
  n135 = call-poly <vilib>:"Read Key.vi"("section"="总磷总氮", "error in (no error)"=w9, "key"="总氮稀释倍数" ("section"), "refnum"=w11) -> ("error out"=w8:errorcluster, "value"=→"总氮稀释倍数":dbl, "refnum out"=w10:T16)  [unwired: 4 in, 1 out]
  n136 = call-by-ref "?"(reference=w40, error in=w38) -> (reference out=w36:refnum<vi>, error out=w37:errorcluster)  [unwired: 12 in]
  n137 = Open VI Reference(type specifier VI Refnum (for type only)=refnum<vi> refnum, vi path=w28, options=128 ("选项")) -> (vi reference=w30:refnum<vi>, error out=w32:errorcluster)  [unwired: 3 in]
  n138 = call "时间延迟2"() -> ("error out"=w12:errorcluster)  [unwired: 11 in]
  n139 = call-by-ref "?"(reference=w30, error in=w32) -> (reference out=w34:refnum<vi>, error out=w33:errorcluster)  [unwired: 12 in]
  n140 = Close Reference(reference=w36, error in (no error)=w37) -> ()  [unwired: 1 out]
  n141 = Close Reference(reference=w34, error in (no error)=w33) -> ()  [unwired: 1 out]
  n142 = call "总磷氨氮MB_api.vi"("STEP"=enum16{"open", "read", "write", "close"}."open", "Error in"=w12) -> ("error out"=w19:errorcluster)  [unwired: 7 in, 2 out]
  n143 = call <vilib>:"Close Config Data.vi"("error in (no error)"=w8, "refnum"=w10) -> ("error out"=w3:errorcluster)  [unwired: 8 in, 1 out]
  n144 = control-ref of="测量模式下拉列表"() -> (w24:refnum<vi>)
  n145 = control-ref of="参数下拉列表"() -> (w25:refnum<vi>)
  n146 = control-ref of="量程下拉列表"() -> (w26:refnum<vi>)
  n147 = control-ref of="量程切换阈值"() -> (w22:refnum<vi>)
  n148 = node-c288(w16) -> ()  [unwired: 1 out]
  n149 = control-ref of="备用系数"() -> (w21:refnum<vi>)
  n150 = control-ref of="公式"() -> (w23:refnum<vi>)
  n151 = Obtain Queue(name (unnamed)="TP" ("名称（未命名）"), element data type=cluster{"命令":string, "data":variant} {"命令"="", "data"=variant}) -> (queue out=w46:refnum<queue>, error out=w47:errorcluster)  [unwired: 3 in, 1 out]
  n152 = while {
    tunnel: w46 -> [w294]
    shift-right: [w295] -> _
    shift-left: T4."待机" -> [w296]
    shift-right: [w292] -> _
    shift-left: u32 0 ("等待时间（毫秒）") -> [w293]
    stop <- FALSE stop-if-true
    n153 = Wait (ms)(milliseconds to wait=u32 1000 ("等待时间（毫秒）")) -> ()  [unwired: 1 out]
    n154 = local read "定时启动"() -> (w297:bool)
    n155 = case shown="真" w297 {
      tunnel: w296 -> [_ w305]
      tunnel: [T4."待机" w304] -> w295
      tunnel: w294 -> [_ w303]
      tunnel: w293 -> [_ w302]
      tunnel: [_ w301] -> w292
      frame False {
      }
      frame True {
        n156 = case shown="\"启动氨氮\"" w305 {
          tunnel: [T4."启动氨氮" w310 w316 w328 w335 w351] -> w304
          tunnel: w303 -> [_ w315 _ w334 _ _]
          tunnel: w302 -> [_ _ _ _ _ w353]
          tunnel: [_ _ _ _ _ w350] -> w301
          frame "待机", Default {
          }
          frame "启动氨氮" {
            n157 = call "总磷氨氮启动命令.vi"("参数"=T17 {"站号"=2, "量程切换"=enum."AUTO", "控制命令"=enum."启动测量", "模式设置"=enum."待机", "测量间隔"=0}) -> ("启动命令"=w308:cluster{"命令":string, "data":variant})  [unwired: 10 in]
            n158 = Enqueue Element(queue=w315, element=w308) -> ()  [unwired: 2 in, 3 out]
            n159 = global read "VAR总磷氨氮全局变量.vi" "状态告警区"() -> (w314:T3)
            n160 = Unbundle By Name(w314) -> ("工作状态"=w313:T7)
            n161 = Not Equal To 0?(x=w313) -> (x != 0?=w312:bool)
            n162 = Select(t=T4."氨氮测量中", s=w312, f=T4."启动氨氮") -> (s? t:f=w310:T4)
          }
          frame "氨氮测量中" {
            n163 = global read "VAR总磷氨氮全局变量.vi" "状态告警区"() -> (w319:T3)
            n164 = Unbundle By Name(w319) -> ("工作状态"=w317:T7, "id"=w318:u16)
            n165 = case shown="\"空闲\"" w317 {
              tunnel: w318 -> [_ w323]
              tunnel: [T4."启动总磷" w322] -> w316
              frame "空闲" {
                n166 = Wait (ms)(milliseconds to wait=u32 5000 ("等待时间（毫秒）")) -> ()  [unwired: 1 out]
              }
              frame Default {
                n167 = case shown="131" w323 {
                  tunnel: [T4."氨氮测量中" T4."总磷测量中"] -> w322
                  frame 76, Default {
                  }
                  frame 131 {
                  }
                }
              }
            }
          }
          frame "启动总磷" {
            n168 = call "总磷氨氮启动命令.vi"("参数"=T17 {"站号"=1, "量程切换"=enum."AUTO", "控制命令"=enum."启动测量", "模式设置"=enum."待机", "测量间隔"=0}) -> ("启动命令"=w327:cluster{"命令":string, "data":variant})  [unwired: 10 in]
            n169 = Enqueue Element(queue=w334, element=w327) -> ()  [unwired: 2 in, 3 out]
            n170 = global read "VAR总磷氨氮全局变量.vi" "状态告警区"() -> (w329:T3)
            n171 = Unbundle By Name(w329) -> ("工作状态"=w330:T7)
            n172 = Not Equal To 0?(x=w330) -> (x != 0?=w331:bool)
            n173 = Select(t=T4."总磷测量中", s=w331, f=T4."启动总磷") -> (s? t:f=w328:T4)
          }
          frame "总磷测量中" {
            n174 = global read "VAR总磷氨氮全局变量.vi" "状态告警区"() -> (w338:T3)
            n175 = Unbundle By Name(w338) -> ("工作状态"=w336:T7, "id"=w337:u16)
            n176 = case shown="\"空闲\"" w336 {
              tunnel: w337 -> [_ w342]
              tunnel: [T4."延时" w341] -> w335
              frame "空闲" {
                n177 = Wait (ms)(milliseconds to wait=u32 5000 ("等待时间（毫秒）")) -> ()  [unwired: 1 out]
              }
              frame Default {
                n178 = case shown="76, 默认" w342 {
                  tunnel: [T4."氨氮测量中" T4."总磷测量中"] -> w341
                  frame 76, Default {
                  }
                  frame 131 {
                  }
                }
              }
            }
          }
          frame "延时" {
            n179 = local read "设置值"() -> (w347:dbl)
            n180 = Increment(x=w353) -> (x+1=w350:u32)
            n181 = Add(x=w347, y=10.0) -> (x+y=w345:dbl)
            n182 = Greater Or Equal?(x=w350, y=w345) -> (x >= y?=w352:bool)
            n183 = Select(t=T4."待机", s=w352, f=T4."延时") -> (s? t:f=w351:T4)
          }
        }
      }
    }
  }
  n184 = while {
    tunnel: w46 -> [w361]
    tunnel: w26 -> [w360]
    tunnel: w25 -> [w359]
    tunnel: w24 -> [w358]
    tunnel: w23 -> [w357]
    tunnel: w22 -> [w356]
    tunnel: w21 -> [w355]
    tunnel: w19 -> [_]
    tunnel: w3 -> [w354]
    stop <- FALSE stop-if-true
    n185 = event shown="[5] \"调试\": 值改变" {
      selector: _ -> [_ _ _ _ _ _ _ _ _ _ _ _ _ _ _ _ _ _]
      dyn-events: _ -> [_ _ _ _ _ _ _ _ _ _ _ _ _ _ _ _ _ _]
      timeout: _ -> [_ _ _ _ _ _ _ _ _ _ _ _ _ _ _ _ _ _]
      tunnel: w361 -> [_ w365 _ w376 w378 _ _ _ _ _ _ _ _ _ _ _ _ _]
      tunnel: w360 -> [_ _ _ _ _ _ _ _ _ _ _ w437 _ w457 w466 _ _ _]
      tunnel: w359 -> [_ _ _ _ _ _ _ _ _ _ _ w435 _ w455 w468 w476 w483 _]
      tunnel: w358 -> [_ _ _ _ _ _ _ _ _ _ _ w436 _ w456 w467 _ _ _]
      tunnel: w357 -> [_ _ _ _ _ _ _ _ _ _ _ w431 _ _ _ _ _ _]
      tunnel: w356 -> [_ _ _ _ _ _ _ _ _ _ _ _ _ w451 _ _ _ _]
      tunnel: w355 -> [_ _ _ _ _ _ _ _ _ _ _ _ _ _ _ w474 _ _]
      tunnel: w354 -> [_ _ _ _ _ _ _ _ _ _ _ _ _ _ _ _ _ _]
      event Timeout {
        n186 = event-data() -> ()  [unwired: 1 in, 3 out]
      }
      event "手动启动": Value Change {
        n187 = event-data() -> ()  [unwired: 1 in, 6 out]
        n188 = call "总磷氨氮启动参数对话框.vi"() -> ("确认"=w363:bool, "元素"=w364:cluster{"命令":string, "data":variant})  [unwired: 10 in]
        n189 = case shown="真" w363 {
          tunnel: w365 -> [_ w367]
          tunnel: w364 -> [_ w366]
          frame False {
          }
          frame True {
            n190 = Enqueue Element(queue=w367, element=w366) -> ()  [unwired: 2 in, 3 out]
          }
        }
      }
      event "定时启动": Mouse Down {
        n191 = event-data() -> ()  [unwired: 1 in, 6 out]
        n192 = call "定时启动对话框.vi"() -> ("设置值"=→"设置值":dbl, "确定输出"=→"定时启动":bool)  [unwired: 10 in]
      }
      event "单步测试": Value Change {
        w371 = u16 1 items=["总磷"=1, "氨氮"=3] ("站号")
        n193 = event-data() -> ()  [unwired: 1 in, 6 out]
        n194 = Bundle("站号"=w371, "总磷氨氮调试"="总磷氨氮调试") -> (w370:cluster{"站号":u16, "总磷氨氮调试":u16[]})  [unwired: 1 in]
        n195 = Bundle By Name(cluster=cluster{"命令":string, "data":variant} {"命令"="", "data"=variant} ("元素"), "命令"="debug", "data"=w370) -> (w373:cluster{"命令":string, "data":variant})
        n196 = Enqueue Element(queue=w376, element=w373) -> ()  [unwired: 2 in, 3 out]
      }
      event "停止": Value Change {
        n197 = event-data() -> ()  [unwired: 1 in, 6 out]
        n198 = Enqueue Element(queue=w378, element=cluster{"命令":string, "data":variant} {"命令"="启动", "data"=variant(cluster{"站号":u16, "控制命令输出":u16[]} {"站号"=1, "控制命令输出"=[2816]})} ("元素")) -> ()  [unwired: 2 in, 3 out]
      }
      event "调试": Value Change {
        n199 = event-data() -> ()  [unwired: 1 in, 6 out]
        n200 = property on="窗格" class="Pane"("Origin"=T5 {"Horizontal"=0, "Vertical"=528} ("原点")) -> ()  [unwired: 2 in, 2 out]
      }
      event "设置 2": Value Change {
        n201 = event-data() -> ()  [unwired: 1 in, 6 out]
        n202 = property on="窗格" class="Pane"("Origin"=T5 {"Horizontal"=0, "Vertical"=1256} ("原点")) -> ()  [unwired: 2 in, 2 out]
      }
      event "返回", "返回 2": Value Change {
        n203 = event-data() -> ()  [unwired: 1 in, 6 out]
        n204 = property on="窗格" class="Pane"("Origin"=T5 {"Horizontal"=0, "Vertical"=0} ("原点")) -> ()  [unwired: 2 in, 2 out]
      }
      event "标液浓度1", "测量吸光度1", "测量吸光度2", "标液浓度2", "测量吸光度3", "标液浓度3", "测量吸光度4", "标液浓度4", "测量吸光度5", "标液浓度5", "样品1启用", "样品3启用", "样品4启用", "样品5启用", "样品2启用", "模型", "method", "精度": Value Change {
        n205 = event-data() -> ()  [unwired: 1 in, 6 out]
        n206 = Replace Array Subset(array=dbl[] [0.0, 0.0, 0.0, 0.0, 0.0] ("数组"), new element #1="标液浓度1", new element #2="标液浓度2", new element #3="标液浓度3", new element #4="标液浓度4", new element #5="标液浓度5") -> (w388:dbl[])  [unwired: 5 in]
        n207 = Replace Array Subset(array=dbl[] [0.0, 0.0, 0.0, 0.0, 0.0] ("数组"), new element #1="测量吸光度1", new element #2="测量吸光度2", new element #3="测量吸光度3", new element #4="测量吸光度4", new element #5="测量吸光度5") -> (w387:dbl[])  [unwired: 5 in]
        n208 = Replace Array Subset(array=bool[] [FALSE, FALSE, FALSE, FALSE, FALSE] ("数组"), new element #1="样品1启用", new element #2="样品2启用", new element #3="样品3启用", new element #4="样品4启用", new element #5="样品5启用") -> (w386:bool[])  [unwired: 5 in]
        n209 = call "线性公式.vi"("精度"="精度", "模型"="模型", "method"="method", "启用"=w386, "监测浓度"=w387, "标液浓度"=w388) -> ("XY图"=→"XY图":cluster{"X Values":dbl[], "Y Values":dbl[]}[], "r^2"=→"r^2":dbl, "拟合方程"=→"拟合公式":string)  [unwired: 3 in]
      }
      event "样品1 F0", "样品1 F1", "样品2 F1", "样品2 F0", "样品3 F1", "样品3 F0", "样品4 F0", "样品4 F1", "样品5 F1", "样品5 F0": Value Change {
        n210 = event-data() -> ()  [unwired: 1 in, 6 out]
        n211 = formula code="E=log(F0/F1);"("F0"="样品5 F0", "F1"="样品5 F1") -> ("E"=w423:dbl)
        n212 = formula code="E=log(F0/F1);"("F0"="样品4 F0", "F1"="样品4 F1") -> ("E"=w422:dbl)
        n213 = formula code="E=log(F0/F1);"("F0"="样品3 F0", "F1"="样品3 F1") -> ("E"=w421:dbl)
        n214 = formula code="E=log(F0/F1);"("F0"="样品2 F0", "F1"="样品2 F1") -> ("E"=w420:dbl)
        n215 = formula code="E=log(F0/F1);"("F0"="样品1 F0", "F1"="样品1 F1") -> ("E"=w419:dbl)
        n216 = property on="测量吸光度5" class="DigNum (严格)"("Val(Sgnl)"=w423) -> ()  [unwired: 2 in, 2 out]
        n217 = property on="测量吸光度4" class="DigNum (严格)"("Val(Sgnl)"=w422) -> ()  [unwired: 2 in, 2 out]
        n218 = property on="测量吸光度3" class="DigNum (严格)"("Val(Sgnl)"=w421) -> ()  [unwired: 2 in, 2 out]
        n219 = property on="测量吸光度2" class="DigNum (严格)"("Val(Sgnl)"=w420) -> ()  [unwired: 2 in, 2 out]
        n220 = property on="测量吸光度1" class="DigNum (严格)"("Val(Sgnl)"=w419) -> ()  [unwired: 2 in, 2 out]
      }
      event "标液浓度1", "标液浓度2", "标液浓度3", "标液浓度4", "标液浓度5", "样品1 F0", "样品1 F1", "样品2 F1", "样品2 F0", "样品3 F1", "样品3 F0", "样品4 F0", "样品4 F1", "样品5 F0", "样品5 F1", "精度", "公式.X^2", "公式.X", "公式.b", "量程切换阈值.阈值", "量程切换阈值.标液浓度", "备用系数.量程上限", "备用系数.量程下限", "备用系数.检出限", "备用系数.精度", "总氮稀释倍数", "测量吸光度1", "测量吸光度2", "测量吸光度3", "测量吸光度4", "测量吸光度5": Mouse Down {
        n221 = event-data() -> ("CtlRef"=w427:refnum<vi>)  [unwired: 1 in, 5 out]
        n222 = property class="DigNum (严格)"(reference=w427) -> (reference out=w425:refnum<vi>, "Value"=w426:dbl)  [unwired: 1 in, 1 out]
        n223 = call "数字键盘.vi"("OldNumber"=w426) -> ("NewNumber"=w424:sgl)
        n224 = property class="DigNum (严格)"(reference=w425, "Val(Sgnl)"=w424) -> ()  [unwired: 1 in, 2 out]
      }
      event "读公式": Value Change {
        n225 = event-data() -> ()  [unwired: 1 in, 6 out]
        n226 = property class="Enum (严格)"(reference=w435) -> ("Value"=w434:enum16{"总磷", "总氮"})  [unwired: 1 in, 2 out]
        n227 = property class="Enum (严格)"(reference=w436) -> ("Value"=w433:enum16{"水样测量", "空白核查", "跨度核查", "标样核查", "加标回收"})  [unwired: 1 in, 2 out]
        n228 = property class="Enum (严格)"(reference=w437) -> ("Value"=w432:enum16{"低量程", "高量程"})  [unwired: 1 in, 2 out]
        n229 = call "总磷氨氮公式读取.vi"("量程"=w432, "测量模式"=w433, "测量参数"=w434) -> ("error out"=w429:errorcluster, "公式"=w430:cluster{"X^2":dbl, "X":dbl, "b":dbl})  [unwired: 7 in]
        n230 = property class="Clust (严格)"(reference=w431, "Value"=w430) -> ()  [unwired: 1 in, 2 out]
        n231 = case shown="错误" w429 {
          tunnel: ["读取成功" ("消息") "读取失败" ("消息")] -> w428
          frame No Error {
          }
          frame Error {
          }
        }
        n232 = One Button Dialog(message=w428) -> ()  [unwired: 1 in, 1 out]
      }
      event "写公式": Value Change {
        n233 = event-data() -> ()  [unwired: 1 in, 6 out]
        n234 = call "总磷氨氮公式写入.vi"("公式"="公式", "量程"="量程下拉列表", "测量模式"="测量模式下拉列表", "测量参数"="参数下拉列表") -> ("error out"=w442:errorcluster)  [unwired: 7 in]
        n235 = case shown="无错误" w442 {
          tunnel: ["写入成功" ("消息") "写入失败" ("消息")] -> w443
          frame No Error {
          }
          frame Error {
          }
        }
        n236 = One Button Dialog(message=w443) -> ()  [unwired: 1 in, 1 out]
      }
      event "量程切换阈值读取": Value Change {
        n237 = event-data() -> ()  [unwired: 1 in, 6 out]
        n238 = property class="Enum (严格)"(reference=w455) -> ("Value"=w454:enum16{"总磷", "总氮"})  [unwired: 1 in, 2 out]
        n239 = property class="Enum (严格)"(reference=w456) -> ("Value"=w453:enum16{"水样测量", "空白核查", "跨度核查", "标样核查", "加标回收"})  [unwired: 1 in, 2 out]
        n240 = property class="Enum (严格)"(reference=w457) -> ("Value"=w452:enum16{"低量程", "高量程"})  [unwired: 1 in, 2 out]
        n241 = call "总磷氨氮量程读取.vi"("量程"=w452, "测量模式"=w453, "测量参数"=w454) -> ("error out"=w448:errorcluster, "量程切换阈值"=w450:cluster{"阈值":dbl, "标液浓度":dbl})  [unwired: 7 in]
        n242 = property class="Clust (严格)"(reference=w451, "Value"=w450) -> ()  [unwired: 1 in, 2 out]
        n243 = case shown="错误" w448 {
          tunnel: ["读取成功" ("消息") "读取失败" ("消息")] -> w449
          frame No Error {
          }
          frame Error {
          }
        }
        n244 = One Button Dialog(message=w449) -> ()  [unwired: 1 in, 1 out]
      }
      event "量程切换阈值写入": Value Change {
        n245 = event-data() -> ()  [unwired: 1 in, 6 out]
        n246 = property class="Enum (严格)"(reference=w468) -> ("Value"=w465:enum16{"总磷", "总氮"})  [unwired: 1 in, 2 out]
        n247 = property class="Enum (严格)"(reference=w467) -> ("Value"=w464:enum16{"水样测量", "空白核查", "跨度核查", "标样核查", "加标回收"})  [unwired: 1 in, 2 out]
        n248 = property class="Enum (严格)"(reference=w466) -> ("Value"=w463:enum16{"低量程", "高量程"})  [unwired: 1 in, 2 out]
        n249 = call "总磷氨氮量程写入.vi"("量程切换阈值"="量程切换阈值", "量程"=w463, "测量模式"=w464, "测量参数"=w465) -> ("error out"=w460:errorcluster)  [unwired: 7 in]
        n250 = case shown="无错误" w460 {
          tunnel: ["写入成功" ("消息") "写入失败" ("消息")] -> w461
          frame No Error {
          }
          frame Error {
          }
        }
        n251 = One Button Dialog(message=w461) -> ()  [unwired: 1 in, 1 out]
      }
      event "备用系数读取": Value Change {
        n252 = event-data() -> ()  [unwired: 1 in, 6 out]
        n253 = property class="Enum (严格)"(reference=w476) -> ("Value"=w475:enum16{"总磷", "总氮"})  [unwired: 1 in, 2 out]
        n254 = call "总磷氨氮备用系数读取.vi"("测量参数"=w475) -> ("error out"=w471:errorcluster, "备用系数"=w473:T1)  [unwired: 9 in]
        n255 = property class="Clust (严格)"(reference=w474, "Value"=w473) -> ()  [unwired: 1 in, 2 out]
        n256 = case shown="错误" w471 {
          tunnel: ["读取成功" ("消息") "读取失败" ("消息")] -> w472
          frame No Error {
          }
          frame Error {
          }
        }
        n257 = One Button Dialog(message=w472) -> ()  [unwired: 1 in, 1 out]
      }
      event "备用系数写入": Value Change {
        n258 = event-data() -> ()  [unwired: 1 in, 6 out]
        n259 = property class="Enum (严格)"(reference=w483) -> ("Value"=w482:enum16{"总磷", "总氮"})  [unwired: 1 in, 2 out]
        n260 = call "总磷氨氮备用系数写入.vi"("备用系数"="备用系数", "测量参数"=w482) -> ("error out"=w479:errorcluster)  [unwired: 9 in]
        n261 = case shown="无错误" w479 {
          tunnel: ["写入成功" ("消息") "写入失败" ("消息")] -> w480
          frame No Error {
          }
          frame Error {
          }
        }
        n262 = One Button Dialog(message=w480) -> ()  [unwired: 1 in, 1 out]
      }
      event "总氮稀释倍数": Value Change {
        n263 = event-data() -> ()  [unwired: 1 in, 6 out]
        n264 = call <vilib>:"Application Directory.vi"() -> ("Application Directory"=w493:path)
        n265 = Build Path(base path=w493, name or relative path="data\\Set.ini" ("名称或相对路径")) -> (appended path=w495:path)
        n266 = local read "总氮稀释倍数"() -> (w488:dbl)
        n267 = call <vilib>:"Open Config Data.vi"("configuration file path"=w495) -> ("error out"=w490:errorcluster, "refnum"=w492:T16)  [unwired: 8 in, 1 out]
        n268 = global write "VAR总磷氨氮全局变量.vi" "总氮稀释倍数"(w488) -> ()
        n269 = call-poly <vilib>:"Write Key.vi"("section"="总磷总氮", "error in (no error)"=w490, "value"=w488, "key"="总氮稀释倍数" ("section"), "refnum"=w492) -> ("error out"=w489:errorcluster, "refnum out"=w491:T16)  [unwired: 4 in, 1 out]
        n270 = call <vilib>:"Close Config Data.vi"("error in (no error)"=w489, "refnum"=w491) -> ()  [unwired: 8 in, 2 out]
      }
    }
  }
  n271 = while {
    tunnel: w46 -> [w512]
    tunnel: w47 -> [_]
    shift-right: [w504] -> _
    shift-left: enum16{"总磷", "总氮"}."总磷" ("枚举") -> [w506]
    stop <- FALSE stop-if-true
    # "试剂填充 172 \n管路清洗108\n氨氮92\n总磷131\n总磷海水147\n总氮76\n总氮海水92"
    n272 = case shown="\"总氮\", 默认" w506 {
      selector: w506 -> [w521 w523]
      tunnel: [w522 w524] -> w507
      tunnel: [w521 w523] -> w505
      frame "总氮", Default {
        w522 = u16 2 items=["总磷"=1, "总氮"=2] ("站号")
      }
      frame "总磷" {
        w524 = u16 1 items=["总磷"=1, "氨氮"=3] ("站号")
      }
    }
    n273 = Wait (ms)(milliseconds to wait=u32 1000 ("等待时间（毫秒）")) -> ()  [unwired: 1 out]
    n274 = Bundle By Name(cluster=cluster{"命令":string, "data":variant} {"命令"="", "data"=variant} ("元素"), "命令"="读状态告警区", "data"=w507) -> (w514:cluster{"命令":string, "data":variant})
    n275 = global read "VAR总磷氨氮全局变量.vi" "状态告警区"() -> (w496:T3)
    n276 = Unbundle By Name(w496) -> ("系统时间"=w503:timestamp)
    n277 = Enqueue Element(queue=w512, element=w514) -> (queue out=w508:refnum<queue>)  [unwired: 2 in, 2 out]
    n278 = Get Date/Time In Seconds() -> (seconds since 1Jan1904=w502:timestamp)
    n279 = Subtract(x=w502, y=w503) -> (x-y=w501:dbl)
    n280 = Bundle By Name(cluster=cluster{"命令":string, "data":variant} {"命令"="", "data"=variant} ("元素"), "命令"="读测量数据区", "data"=w507) -> (w510:cluster{"命令":string, "data":variant})
    n281 = Absolute Value(x=w501) -> (abs(x)=w500:dbl)
    n282 = Enqueue Element(queue=w508, element=w510) -> (queue out=w497:refnum<queue>)  [unwired: 2 in, 2 out]
    n283 = Greater Or Equal?(x=w500, y=120.0) -> (x >= y?=w498:bool)
    n284 = case shown="真" w498 {
      tunnel: w497 -> [_ w519]
      frame False {
      }
      frame True {
        n285 = call "总磷氨氮启动命令.vi"("参数"=T18 {"站号"=3, "量程切换"=enum."AUTO", "控制命令"=enum."校时", "模式设置"=enum."待机", "测量间隔"=0}) -> ("启动命令"=w518:cluster{"命令":string, "data":variant})  [unwired: 10 in]
        n286 = Enqueue Element(queue=w519, element=w518) -> ()  [unwired: 2 in, 3 out]
      }
    }
    n287 = Increment(x=w505) -> (x+1=w504:enum16{"总磷", "总氮"})
  }
